vi "_JsonFile_GetAttribute.vi"(8 "error in (no error)":errorcluster, 10 "Attribute":string, 11 "Json":path) -> (0 "error out":errorcluster, 1 "Found?":bool, 2 "String":string, 3 "Json (dup)":path)   [LabVIEW 2019, in "lv-apt-json-file.lvlib"]
uses:
  lv-apt-json-file.lvlib
  <vilib>/addons/_JKI.lib/Serialization/JSON/JKI JSON Serialization.lvlib
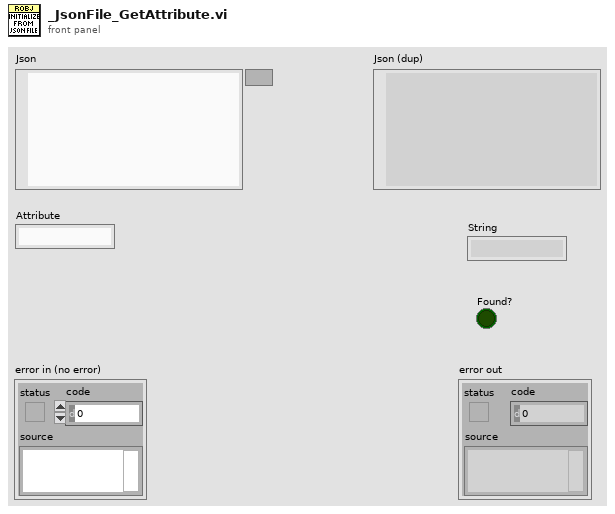
[diagram p1: front panel]
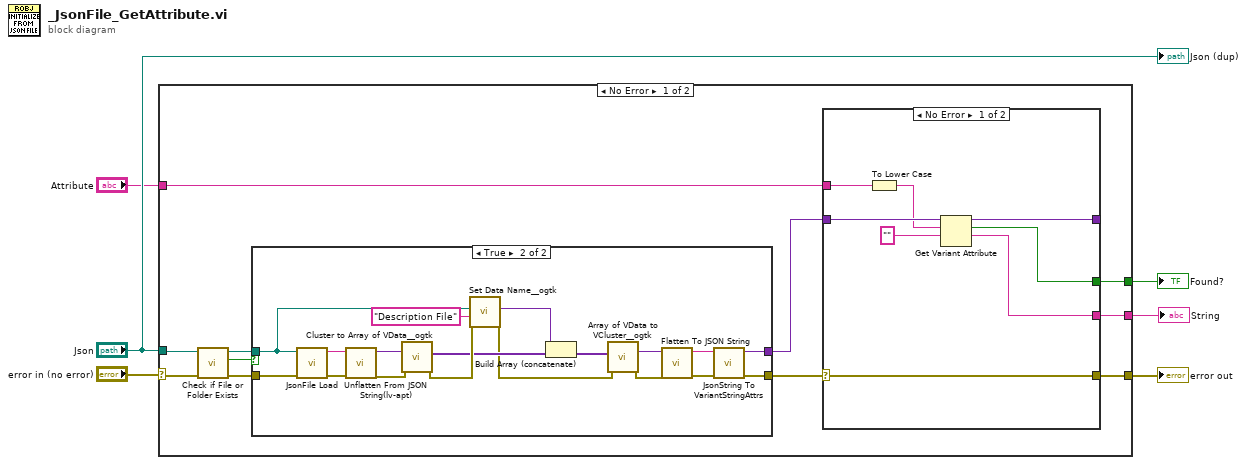
[diagram p0: block diagram]
diagram:
  n1 = case shown="No Error" "error in (no error)" {
    selector: "error in (no error)" -> [w10 w47]
    tunnel: "Json" -> [w17 _]
    tunnel: [w15 w47] -> w5
    tunnel: "Attribute" -> [w13 _]
    tunnel: [w12 _] -> w2
    tunnel: [w11 _] -> w1
    frame No Error {
      n2 = call <vilib>:"Check if File or Folder Exists.vi"("error in (no error)"=w10, "path"=w17) -> ("error out"=w9:errorcluster, "file or folder exists?"=w7:bool, "dup path"=w8:path)  [unwired: 7 in]
      n3 = case shown="True" w7 {
        tunnel: [w18 w22] -> w16
        tunnel: [_ w21] -> w14
        tunnel: w9 -> [w18 w20]
        tunnel: w8 -> [_ w19]
        frame False {
        }
        frame True {
          n4 = call "JsonFile Load.vi"("error in (no error)"=w20, "Path"=w19) -> ("error out"=w34:errorcluster, "Json"=w33:string)  [unwired: 8 in]
          n5 = call "Unflatten From JSON String(lv-apt).vi"("error in (no error)"=w34, "JSON String"=w33) -> ("error out"=w36:errorcluster, "Variant"=w35:variant)  [unwired: 8 in]
          n6 = call <userlib>:"Cluster to Array of VData__ogtk.vi"("error in (no error)"=w36, "Cluster"=w35) -> ("error out"=w31:errorcluster, "Array of VData"=w29:variant[])  [unwired: 8 in]
          n7 = call <userlib>:"Set Data Name__ogtk.vi"("error in (no error)"=w31, "Data Name"="Description File", "Data"=w19) -> ("error out"=w27:errorcluster, "Renamed Data"=w30:variant)  [unwired: 7 in]
          n8 = Build Array (concatenate)(w30, w29) -> (w28:variant[])
          n9 = call <userlib>:"Array of VData to VCluster__ogtk.vi"("error in (no error)"=w27, "Array"=w28) -> ("error out"=w26:errorcluster, "VCluster"=w25:variant)  [unwired: 8 in]
          n10 = call <vilib>:"Flatten To JSON String.vi"("error in (no error)"=w26, "Variant"=w25) -> ("error out"=w23:errorcluster, "JSON String"=w24:string)  [unwired: 8 in]
          n11 = call "JsonString To VariantStringAttrs.vi"("error in (no error)"=w23, "Json"=w24) -> ("error out"=w22:errorcluster, "Variant"=w21:variant)  [unwired: 8 in]
        }
      }
      n12 = case shown="No Error" w16 {
        selector: w16 -> [w38 w46]
        tunnel: w14 -> [w44 w45]
        tunnel: w13 -> [w40 _]
        tunnel: [w43 w45] -> _
        tunnel: [w38 w46] -> w15
        tunnel: [w42 _] -> w12
        tunnel: [w41 _] -> w11
        frame No Error {
          n13 = To Lower Case(string=w40) -> (all lower case string=w39:string)
          n14 = Get Variant Attribute(Variant=w44, name=w39, default value (empty Variant)="") -> (duplicate Variant=w43:variant, found=w42:bool, value=w41:string)  [unwired: 1 in, 1 out]
        }
        frame Error {
        }
      }
    }
    frame Error {
    }
  }
  "error out" <- w5
  "Found?" <- w2
  "String" <- w1
  "Json (dup)" <- "Json"
